vi "SID_DC_blocking.vi"(5 "sampling info":cluster{"Fs":dbl, "#s":i32}={"Fs"=44100.0, "#s"=50}, 9 "R":dbl=0.995, 10 "low pass":dbl=8000.0, 11 "wave in":dbl[](array[numeric])) -> (3 "wave out":dbl[](array[numeric]))   [LabVIEW 2018]
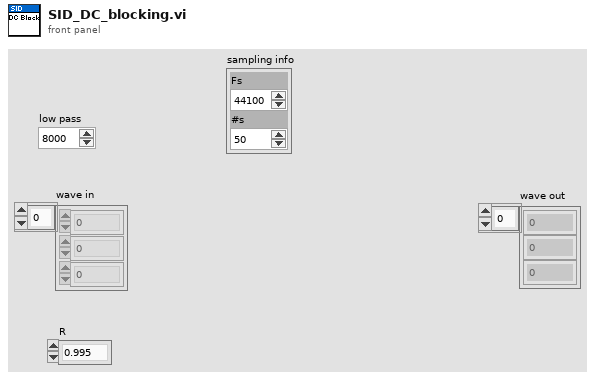
[diagram p1: front panel]
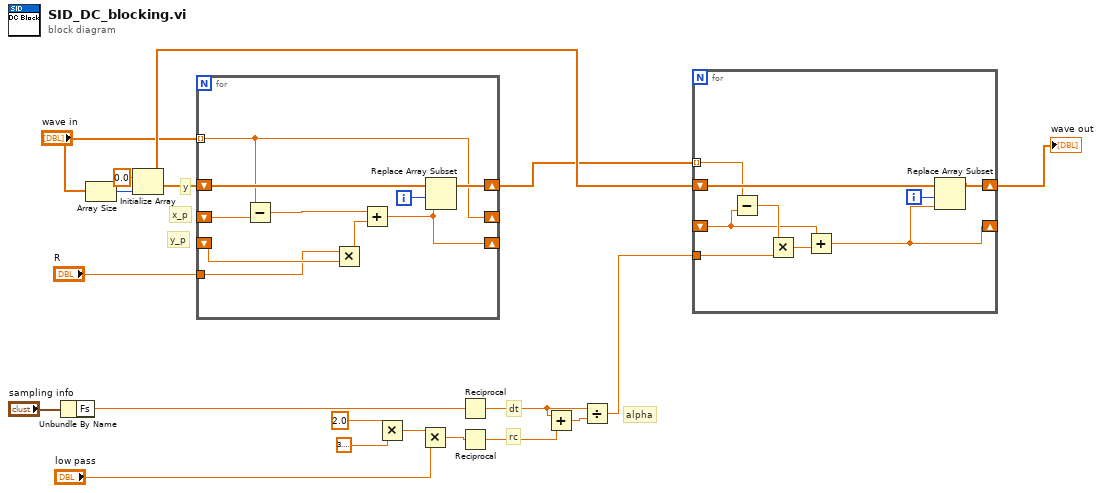
[diagram p0: block diagram]
diagram:
  # "alpha"
  # "dt"
  # "rc"
  # "y"
  # "y_p"
  # "x_p"
  n1 = Unbundle By Name("sampling info") -> ("Fs"=w1:dbl)
  n2 = Array Size(array="wave in") -> (size(s)=w18:i32)
  n3 = Initialize Array(0.0 ("element"), w18) -> (w6:dbl[])
  n4 = for {
    shift-right: [w24] -> w3
    shift-left: w6 -> [w25]
    shift-right: [w22] -> _
    shift-left: _ -> [w28]
    shift-right: [w19] -> _
    shift-left: _ -> [w26]
    tunnel: "wave in" -> [w22] mode=indexing
    tunnel: "R" -> [w21]
    i -> [w23]
    n5 = Subtract(x=w22, y=w28) -> (x-y=w27:dbl)
    n6 = Multiply(x=w21, y=w26) -> (x*y=w20:dbl)
    n7 = Add(x=w27, y=w20) -> (x+y=w19:dbl)
    n8 = Replace Array Subset(array=w25, new element=w19, index=w23) -> (w24:dbl[])
  }
  n9 = Multiply(x=2.0, y=3.141592653589793) -> (x*y=w13:dbl)
  n10 = Multiply(x=w13, y="low pass") -> (x*y=w11:dbl)
  n11 = Reciprocal(x=w1) -> (1/x=w8:dbl)
  n12 = Reciprocal(x=w11) -> (1/x=w10:dbl)
  n13 = Add(x=w8, y=w10) -> (x+y=w9:dbl)
  n14 = Divide(x=w8, y=w9) -> (x/y=w7:dbl)
  n15 = for {
    shift-right: [w37] -> w5
    shift-left: w6 -> [w36]
    tunnel: w7 -> [w34]
    tunnel: w3 -> [w33] mode=indexing
    shift-right: [w29] -> _
    shift-left: _ -> [w30]
    i -> [w35]
    n16 = Subtract(x=w33, y=w30) -> (x-y=w32:dbl)
    n17 = Multiply(x=w32, y=w34) -> (x*y=w31:dbl)
    n18 = Add(x=w30, y=w31) -> (x+y=w29:dbl)
    n19 = Replace Array Subset(array=w36, new element=w29, index=w35) -> (w37:dbl[])
  }
  "wave out" <- w5
